vi "Channel Probe.vi"(2 "channelOp":T1, 3 "data in":refnum<class "EventMessengerPData.lvclass">) -> (1 "data out":refnum<class "EventMessengerPData.lvclass">)   [LabVIEW 2020, in "Event Messenger Priority.lvlib"]
doc: "Displays the status of the channel as the channel is modified by the various endpoints and gives the user ways to pause the application using the channel."
uses:
  Event Messenger Priority.lvlib
  EventMessengerPData.lvclass
  ChannelOp.ctl
panel:
  in  "Details":string="Details"
  in  "Write Count":string="Write Count"
  out "Details":string
  in  "Pause when aborted":bool
  in  "Pause when last element written":bool
  out "Details":string
  in  "Play":bool
  out "Aborted?":bool
  out "Last element written?":bool
  in  "Pause":bool
  # "Details"
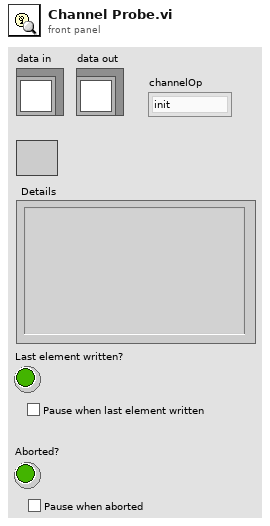
[diagram p1: front panel]
types:
  T1 = typedef "Event Messenger Priority.lvlib/ChannelOp.ctl" = enum16{"init", "write", "register", "replicate", "probe"}
  T2 = enum32{"Invalid", "Standard", "Closed", "Hidden", "Minimized", "Maximized"}
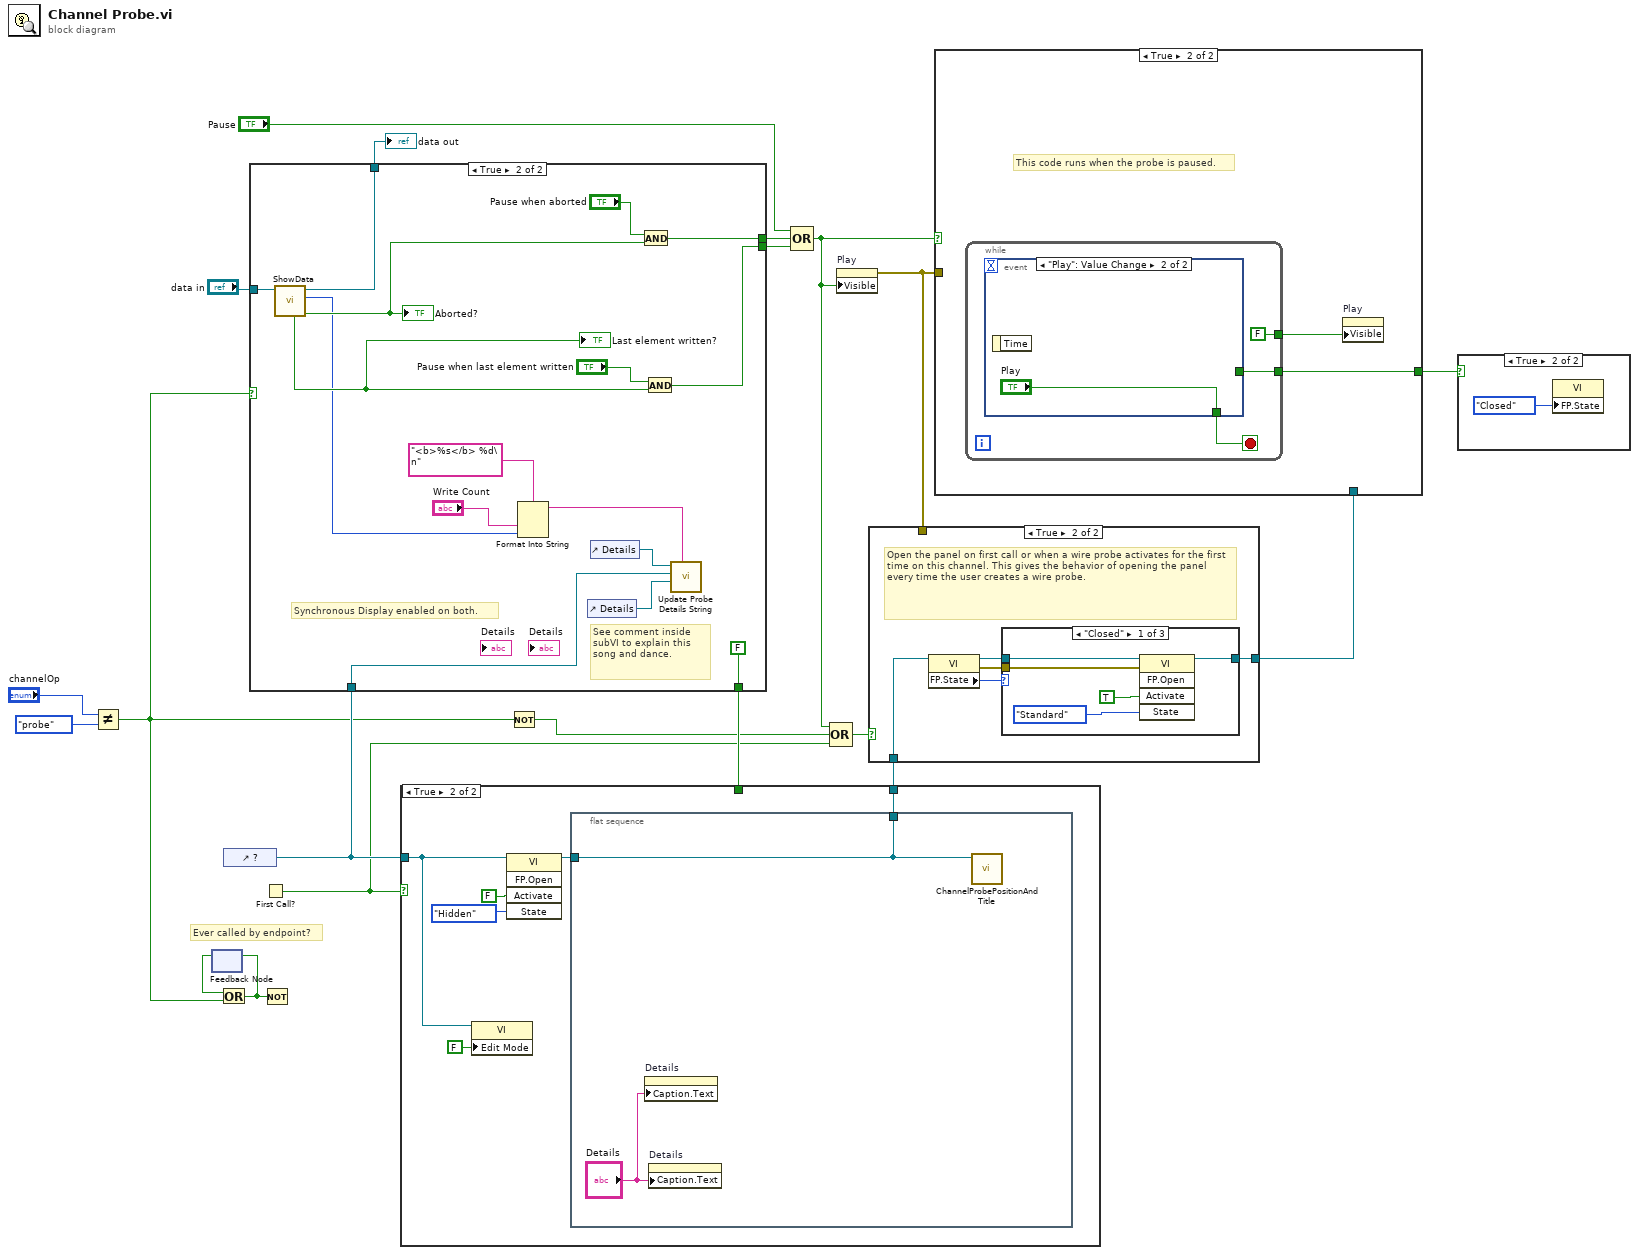
[diagram p0: block diagram]
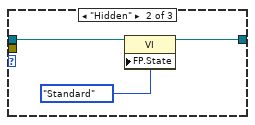
[diagram p3: hidden frame]
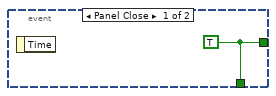
[diagram p8: hidden frame]
diagram:
  # "Ever called by endpoint?"
  n1 = Not Equal?(x="channelOp", y=ChannelOp."probe" ("channelOp")) -> (x != y?=w1:bool)
  n2 = feedback #1() -> (w13:bool)  [unwired: 1 in]
  n3 = Or(x=w13, y=w1) -> (x .or. y?=w12:bool)
  n4 = feedback-in #1(w12) -> ()
  n5 = control-ref of="?"() -> (w14:refnum<vi>)
  n6 = case shown="True" w1 {
    tunnel: "data in" -> [w21 w37]
    tunnel: [_ w34] -> w18
    tunnel: [_ w33] -> w16
    tunnel: [_ FALSE ("always false")] -> w15
    tunnel: w14 -> [_ w31]
    tunnel: [w21 w26] -> w3
    frame False {
    }
    frame True {
      # "See comment inside subVI to explain this song and dance."
      # "Synchronous Display enabled on both."
      n7 = call "ShowData.vi"("data in"=w37) -> ("aborted?"=w24:bool, "write count"=w23:u32, "data out"=w26:refnum<class "EventMessengerPData.lvclass">, "last element?"=w25:bool)  [unwired: 7 in]
      "Last element written?" <- w25
      "Aborted?" <- w24
      n8 = Format Into String(format string="<b>%s</b> %d\n", "Write Count", w23) -> (resulting string=w22:string)  [unwired: 2 in, 1 out]
      n9 = control-ref of="Details"() -> (w32:refnum<vi>)
      n10 = control-ref of="Details"() -> (w30:refnum<vi>)
      n11 = And(x="Pause when aborted", y=w24) -> (x .and. y?=w34:bool)
      n12 = And(x="Pause when last element written", y=w25) -> (x .and. y?=w33:bool)
      n13 = call <resource>:"Update Probe Details String.vi"("String"=w22, "Details 1"=w32, "VI Reference"=w31, "Details 2"=w30) -> ()  [unwired: 8 in]
    }
  }
  "data out" <- w3
  n14 = First Call?() -> (First Call?: T/F=w5:bool)
  n15 = Not(x=w12) -> ()  [unwired: 1 out]
  n16 = case shown="True" w5 {
    tunnel: [w38 w44] -> w10
    tunnel: w14 -> [w38 w40]
    tunnel: w15 -> [_ _]
    frame False {
    }
    frame True {
      n17 = property class="VI"(reference=w40, "Edit Mode"=FALSE ("Edit Mode On Open")) -> ()  [unwired: 1 in, 2 out]
      n18 = invoke class="VI" method="FP.Open"(reference=w40, "Activate"=FALSE ("Activate?"), "State"=T2."Hidden") -> (reference out=w41:refnum<vi>)  [unwired: 2 in, 4 out]
      n19 = flat-sequence {
        tunnel: [w45] -> w44
        tunnel: w41 -> [w45]
        frame #0 {
          n20 = property on="Details" class="Str"("Caption.Text"="Details") -> ()  [unwired: 2 in, 2 out]
          n21 = property on="Details" class="Str"("Caption.Text"="Details") -> ()  [unwired: 2 in, 2 out]
          n22 = call <resource>:"ChannelProbePositionAndTitle.vi"("VI in"=w45) -> ()  [unwired: 9 in, 2 out]
        }
      }
    }
  }
  n23 = Not(x=w1) -> (.not. x?=w6:bool)
  n24 = Compound Arithmetic op=OR("Pause", w18, w16) -> (w2:bool)
  n25 = Compound Arithmetic op=OR(w2, w6, w5) -> (w4:bool)
  n26 = property on="Play" class="Bool"("Visible"=w2) -> (error out=w9:errorcluster)  [unwired: 2 in, 1 out]
  n27 = case shown="True" w4 {
    tunnel: [w47 w49] -> w11
    tunnel: w10 -> [w47 w48]
    tunnel: w9 -> [_ _]
    frame False {
    }
    frame True {
      # "Open the panel on first call or when a wire probe activates for the first time on this channel. This gives the behavior of opening the panel every time the user creates a wire probe."
      n28 = property class="VI"(reference=w48) -> (reference out=w50:refnum<vi>, error out=w51:errorcluster, "FP.State"=w52:T2)  [unwired: 1 in]
      n29 = case shown="\"Closed\"" w52 {
        tunnel: w51 -> [w56 _ _]
        tunnel: w50 -> [w57 w60 w61]
        tunnel: [w53 w59 w61] -> w49
        frame "Closed" {
          n30 = invoke class="VI" method="FP.Open"(reference=w57, error in=w56, "Activate"=TRUE ("Activate?"), "State"=T2."Standard") -> (reference out=w53:refnum<vi>)  [unwired: 1 in, 4 out]
        }
        frame "Hidden" {
          n31 = property class="VI"(reference=w60, "FP.State"=T2."Standard" ("Front Panel Window:State")) -> (reference out=w59:refnum<vi>)  [unwired: 1 in, 1 out]
        }
        frame Default {
        }
      }
    }
  }
  n32 = case shown="True" w2 {
    tunnel: w11 -> [_ _]
    tunnel: [_ w63] -> w20
    tunnel: w9 -> [_ _]
    frame False {
    }
    frame True {
      # "This code runs when the probe is paused."
      n33 = while {
        tunnel: [w66] -> w63
        tunnel: [FALSE ("Visible")] -> w62
        stop <- w65 stop-if-true
        n34 = event shown="[1] \"Play\": Value Change" {
          selector: _ -> [_ _]
          dyn-events: _ -> [_ _]
          timeout: _ -> [_ _]
          tunnel: [w67 _] -> w66
          tunnel: [w67 "Play"] -> w65
          event Panel Close {
            w67 = TRUE
            n35 = event-data() -> ()  [unwired: 1 in, 1 out]
          }
          event "Play": Value Change {
            n36 = event-data() -> ()  [unwired: 1 in, 1 out]
          }
        }
      }
      n37 = property on="Play" class="Bool"("Visible"=w62) -> ()  [unwired: 2 in, 2 out]
    }
  }
  n38 = case shown="True" w20 {
    frame False {
    }
    frame True {
      n39 = property class="VI"("FP.State"=T2."Closed" ("Front Panel Window:State")) -> ()  [unwired: 2 in, 2 out]
    }
  }
